vi "Utility - Configuration File Generator.vi"() -> ()   [LabVIEW 2013]
uses:
  controls/TDMS Properties.ctl
  controls/Acquisition and Logging Configuration.ctl
  <vilib>/Utility/xml.llb/Write to XML File(string).vi
panel:
  in  "Enable Time Trigger":bool
  in  "Enable RMS Trigger":bool=TRUE
  in  "Log Continuously":bool
  in  "TDMS Properties":T1[](array[typedef])=[{"Name"="Enterprise", "Value"="[CompanyName]"}, {"Name"="Author", "Value"="[DeveloperName]"}, {"Name"="Operator", "Value"="[OperatorName]"}, {"Name"="TestSystem", "Value"="[SystemName]"}, {"Name"="Site", "Value"="[Location]"}, {"Name"="Line", "Value"="[Line]"}, {"Name"="Machine", "Value"="[MachineName]"}, {"Name"="Description", "Value"="[Description]"}]
  in  "Trigger - Time (Minute)":i32=30
  in  "Trigger - Channel":i32
  in  "Trigger - RMS Value":dbl=2.0
  in  "Channel Names":string[](array[string])=["Dev1/ai0", "Dev1/ai1", "Dev1/ai2", "Dev1/ai3"]
  in  "Channel Scale Array":dbl[](array[numeric])=[1.0, 1.0, 1.0, 1.0]
  in  "Number of Channels":i32=4
  in  "Data File Name":string="DAQ_Data"
  in  "Number of Reads to Save":i32=20
  in  "Samples per Read":i32=1000
  in  "Data Rate (Hz)":dbl=1000.0
  # "Instructions: Populate the controls below with desired values, then run the VI to generate a 'Config.xml' file in the root folder of your project.  \n\nNote:  Once you have generated the Config.xml file, you will need to copy it to the root folder of your RT Target."
  # "Acquisition"
  # "Channels"
  # "Logging"
  # "Trigger"
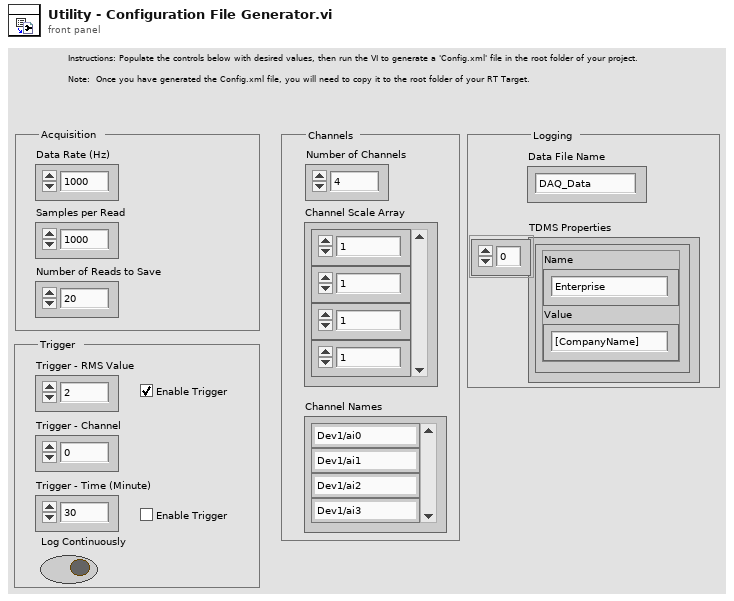
[diagram p1: front panel]
types:
  T1 = typedef "TDMS Properties.ctl" = cluster{"Name":string, "Value":string}
  T2 = typedef "Acquisition and Logging Configuration.ctl" = cluster{"Data Rate (Hz)":dbl, "Samples per Read":i32, "Number of Reads to Save":i32, "Data File Name":string, "TDMS Properties":T1[], "Number of Channels":i32, "Channel Scale Array":dbl[], "Channel Names":string[], "Trigger - RMS Value":dbl, "Trigger - Channel":i32, "Trigger - Time (Minute)":i32, "Enable RMS Trigger":bool, "Enable Time Trigger":bool, "Always Log":bool}
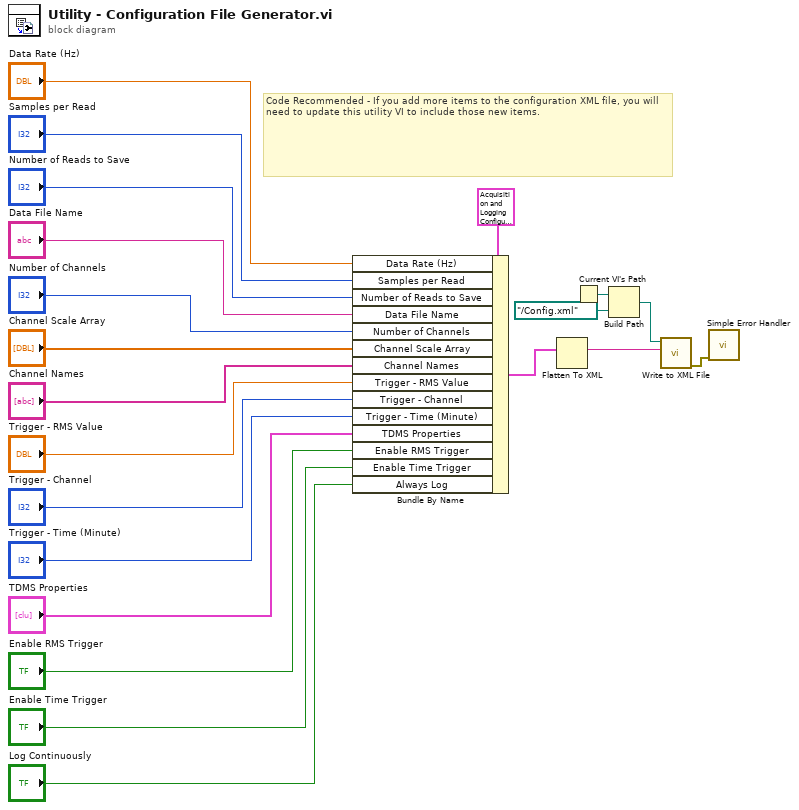
[diagram p0: block diagram]
diagram:
  # "Code Recommended - If you add more items to the configuration XML file, you will need to update this utility VI to include those new items."
  n1 = Bundle By Name(cluster=T2 {"Data Rate (Hz)"=1.0, "Samples per Read"=0, "Number of Reads to Save"=0, "Data File Name"="", "TDMS Properties"=[], "Number of Channels"=0, "Channel Scale Array"=[0.0, 0.0, 0.0, 0.0], "Channel Names"=[], "Trigger - RMS Value"=0.0, "Trigger - Channel"=0, "Trigger - Time (Minute)"=0, "Enable RMS Trigger"=FALSE, "Enable Time Trigger"=FALSE, "Always Log"=FALSE} ("Acquisition and Logging Configuration"), "Data Rate (Hz)"="Data Rate (Hz)", "Samples per Read"="Samples per Read", "Number of Reads to Save"="Number of Reads to Save", "Data File Name"="Data File Name", "Number of Channels"="Number of Channels", "Channel Scale Array"="Channel Scale Array", "Channel Names"="Channel Names", "Trigger - RMS Value"="Trigger - RMS Value", "Trigger - Channel"="Trigger - Channel", "Trigger - Time (Minute)"="Trigger - Time (Minute)", "TDMS Properties"="TDMS Properties", "Enable RMS Trigger"="Enable RMS Trigger", "Enable Time Trigger"="Enable Time Trigger", "Always Log"="Log Continuously") -> (w20:T2)
  n2 = Flatten To XML(anything=w20) -> (xml string=w19:string)
  n3 = Current VI's Path() -> (path=w18:path)
  n4 = Build Path(base path=w18, name or relative path=path "../Config.xml") -> (appended path=w16:path)
  n5 = call-poly <vilib>:"Write to XML File.vi"("XML Input"=w19, "XML File Path"=w16) -> ("error out"=w15:errorcluster)  [unwired: 7 in, 2 out]
  n6 = call <vilib>:"Simple Error Handler.vi"("error in (no error)"=w15) -> ()  [unwired: 4 in, 5 out]
